vi "get_switch.vi"(8 "error in (no error)":errorcluster, 10 "channel":u16, 11 "SwitchBoxConrad in":refnum<class "SwitchBoxConrad.lvclass">) -> (0 "error out":errorcluster, 1 "String":string, 2 "actual switch state":bool, 3 "SwitchBoxConrad out":refnum<class "SwitchBoxConrad.lvclass">)   [LabVIEW 2018, in "SwitchBoxConrad.lvclass"]
doc: "get state of a specific switch channel from the actual instrument"
uses:
  SwitchBoxConrad.lvclass
  instrument.lvclass
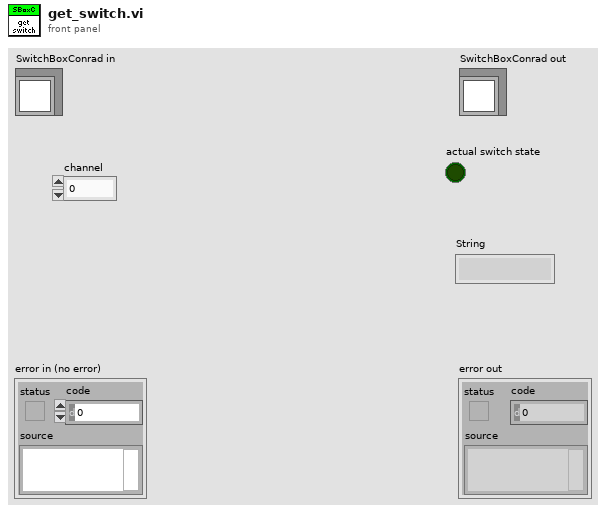
[diagram p1: front panel]
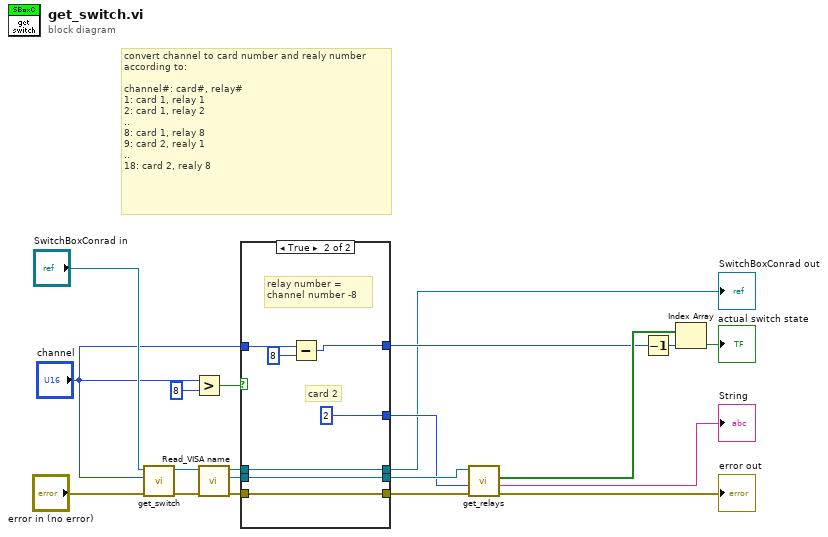
[diagram p0: block diagram]
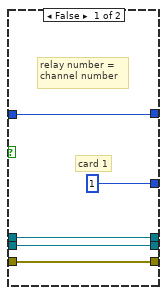
[diagram p2: hidden frame]
diagram:
  # "convert channel to card number and realy number\naccording to:\n\nchannel#: card#, relay#\n1: card 1, relay 1\n2: card 1, relay 2\n..\n8: card 1, relay 8\n9: card 2, realy 1\n..\n18: card 2, realy 8"
  n1 = call-parent "get_switch.vi"("error in (no error)"="error in (no error)", "channel"="channel", "instrument in"="SwitchBoxConrad in") -> ("error out"=w13:errorcluster, "instrument out"=w14:refnum<class "SwitchBoxConrad.lvclass">)  [unwired: 5 in, 2 out]
  n2 = Greater?(x="channel", y=u16 8) -> (0:w18:bool)
  n3 = call-dynamic "Read_VISA name.vi"("error in (no error)"=w13, "instrument in"=w14) -> ("error out"=w16:errorcluster, "VISA resource name"=w15:refnum<visa-resource-name>, "instrument out"=w17:refnum<class "SwitchBoxConrad.lvclass">)  [unwired: 7 in]
  n4 = case shown="True" w18 {
    tunnel: "channel" -> [w21 w30]
    tunnel: w17 -> [w25 w32]
    tunnel: w16 -> [w24 w31]
    tunnel: [w25 w32] -> w3
    tunnel: [w24 w31] -> w9
    tunnel: [u8 1 u8 2] -> w8
    tunnel: [w21 w27] -> w5
    tunnel: w15 -> [w22 w28]
    tunnel: [w22 w28] -> w10
    frame False {
      # "relay number =\nchannel number"
      # "card 1"
    }
    frame True {
      # "relay number =\nchannel number -8"
      # "card 2"
      n5 = Subtract(x=w30, y=u16 8) -> (x-y=w27:u16)
    }
  }
  "SwitchBoxConrad out" <- w3
  n6 = call "get_relays.vi"("error in (no error)"=w9, "card address"=w8, "VISA Refnum in"=w10) -> ("error out"=→"error out":errorcluster, "return string"=→"String":string, "boolian array out"=w7:bool[])  [unwired: 5 in, 1 out]
  n7 = Decrement(x=w5) -> (x-1=w6:u16)
  n8 = Index Array(array=w7, index=w6) -> (element=→"actual switch state":bool)
